vi "Decorate.vi"(10 "Event jettl":refnum<class "Event jettl.lvclass">, 11 "Hello World Event in":refnum<class "Hello World Event.lvclass">) -> (3 "Hello World Event out":refnum<class "Hello World Event.lvclass">)   [LabVIEW 2021, in "Hello World Event.lvlib" / "Hello World Event.lvclass"]
uses:
  Hello World Event.lvclass
  Hello World Event.lvclass/Hello World Event.ctl
  jettl/Event jettl/Event jettl.lvclass
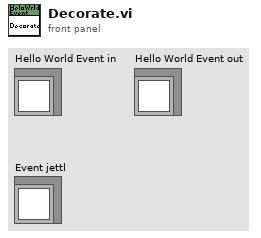
[diagram p1: front panel]
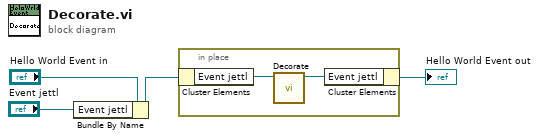
[diagram p0: block diagram]
diagram:
  n1 = Bundle By Name(cluster="Hello World Event in", "Event jettl"="Event jettl") -> (w2:refnum<class "Hello World Event.lvclass">)
  n2 = in-place {
    n3 = in-place-cluster #1(w2) -> ("Event jettl"=w6:refnum<class "Event jettl.lvclass">)
    n4 = call-dynamic "Decorate.vi"("Event jettl in"=w6) -> ("Event jettl out"=w5:refnum<class "Event jettl.lvclass">)  [unwired: 10 in]
    n5 = in-place-cluster #1("Event jettl"=w5) -> (→"Hello World Event out":refnum<class "Hello World Event.lvclass">)
  }
